vi "LabVIEW OPC UA Client.vi"() -> ()   [LabVIEW 2020]
uses:
  <vilib>/OPCUA/NI OPC UA Client.lvlib
  <vilib>/OPCUA/NI OPC UA Utility.lvlib
  <vilib>/OPCUA/controls/Write Status.ctl
  <vilib>/OPCUA/controls/NodeId.ctl
  <vilib>/OPCUA/client/Multiple Write Double.vi
  <vilib>/OPCUA/client/Multiple Read Double.vi
panel:
  out "DateTime":string
  out "Status":u32(ring) items=["Good", "Good_SubscriptionTransferred", "Good_CompletesAsynchronously", "Good_Overload", "Good_Clamped", "Good_LocalOverride", "Good_EntryInserted", "Good_EntryReplaced", "Good_NoData", "Good_MoreData", "Good_CommunicationEvent", "Good_ShutdownEvent", "Good_CallAgain", "Good_NonCriticalTimeout", "Good_ResultsMayBeIncomplete", "Good_DataIgnored", "Uncertain", "Uncertain_ReferenceOutOfServer", "Uncertain_NoCommunicationLastUsableValue", "Uncertain_LastUsableValue", "Uncertain_SubstituteValue", "Uncertain_InitialValue", "Uncertain_SensorNotAccurate", "Uncertain_EngineeringUnitsExceeded", "Uncertain_SubNormal", "Uncertain_DataSubNormal", "Uncertain_ReferenceNotDeleted", "Uncertain_NotAllNodesAvailable", "Bad", "Bad_UnexpectedError", "Bad_InternalError", "Bad_OutOfMemory", "Bad_ResourceUnavailable", "Bad_CommunicationError", "Bad_EncodingError", "Bad_DecodingError", "Bad_EncodingLimitsExceeded", "Bad_UnknownResponse", "Bad_Timeout", "Bad_ServiceUnsupported", "Bad_Shutdown", "Bad_ServerNotConnected", "Bad_ServerHalted", "Bad_NothingToDo", "Bad_TooManyOperations", "Bad_DataTypeIdUnknown", "Bad_CertificateInvalid", "Bad_SecurityChecksFailed", "Bad_CertificateTimeInvalid", "Bad_CertificateIssuerTimeInvalid", "Bad_CertificateHostNameInvalid", "Bad_CertificateUriInvalid", "Bad_CertificateUseNotAllowed", "Bad_CertificateIssuerUseNotAllowed", "Bad_CertificateUntrusted", "Bad_CertificateRevocationUnknown", "Bad_CertificateIssuerRevocationUnknown", "Bad_CertificateRevoked", "Bad_CertificateIssuerRevoked", "Bad_UserAccessDenied", "Bad_IdentityTokenInvalid", "Bad_IdentityTokenRejected", "Bad_SecureChannelIdInvalid", "Bad_InvalidTimestamp", "Bad_NonceInvalid", "Bad_SessionIdInvalid", "Bad_SessionClosed", "Bad_SessionNotActivated", "Bad_SubscriptionIdInvalid", "Bad_RequestHeaderInvalid", "Bad_TimestampsToReturnInvalid", "Bad_RequestCancelledByClient", "Bad_NoCommunication", "Bad_WaitingForInitialData", "Bad_NodeIdInvalid", "Bad_NodeIdUnknown", "Bad_AttributeIdInvalid", "Bad_IndexRangeInvalid", "Bad_IndexRangeNoData", "Bad_DataEncodingInvalid", "Bad_DataEncodingUnsupported", "Bad_NotReadable", "Bad_NotWritable", "Bad_OutOfRange", "Bad_NotSupported", "Bad_NotFound", "Bad_ObjectDeleted", "Bad_NotImplemented", "Bad_MonitoringModeInvalid", "Bad_MonitoredItemIdInvalid", "Bad_MonitoredItemFilterInvalid", "Bad_MonitoredItemFilterUnsupported", "Bad_FilterNotAllowed", "Bad_StructureMissing", "Bad_EventFilterInvalid", "Bad_ContentFilterInvalid", "Bad_FilterOperandInvalid", "Bad_ContinuationPointInvalid", "Bad_NoContinuationPoints", "Bad_ReferenceTypeIdInvalid", "Bad_BrowseDirectionInvalid", "Bad_NodeNotInView", "Bad_ServerUriInvalid", "Bad_ServerNameMissing", "Bad_DiscoveryUrlMissing", "Bad_SempahoreFileMissing", "Bad_RequestTypeInvalid", "Bad_SecurityModeRejected", "Bad_SecurityPolicyRejected", "Bad_TooManySessions", "Bad_UserSignatureInvalid", "Bad_ApplicationSignatureInvalid", "Bad_NoValidCertificates", "Bad_RequestCancelledByRequest", "Bad_ParentNodeIdInvalid", "Bad_ReferenceNotAllowed", "Bad_NodeIdRejected", "Bad_NodeIdExists", "Bad_NodeClassInvalid", "Bad_BrowseNameInvalid", "Bad_BrowseNameDuplicated", "Bad_NodeAttributesInvalid", "Bad_TypeDefinitionInvalid", "Bad_SourceNodeIdInvalid", "Bad_TargetNodeIdInvalid", "Bad_DuplicateReferenceNotAllowed", "Bad_InvalidSelfReference", "Bad_ReferenceLocalOnly", "Bad_NoDeleteRights", "Bad_ServerIndexInvalid", "Bad_ViewIdUnknown", "Bad_TooManyMatches", "Bad_QueryTooComplex", "Bad_NoMatch", "Bad_MaxAgeInvalid", "Bad_HistoryOperationInvalid", "Bad_HistoryOperationUnsupported", "Bad_WriteNotSupported", "Bad_TypeMismatch", "Bad_MethodInvalid", "Bad_ArgumentsMissing", "Bad_TooManySubscriptions", "Bad_TooManyPublishRequests", "Bad_NoSubscription", "Bad_SequenceNumberUnknown", "Bad_MessageNotAvailable", "Bad_InsufficientClientProfile", "Bad_TcpServerTooBusy", "Bad_TcpMessageTypeInvalid", "Bad_TcpSecureChannelUnknown", "Bad_TcpMessageTooLarge", "Bad_TcpNotEnoughResources", "Bad_TcpInternalError", "Bad_TcpEndpointUrlInvalid", "Bad_RequestInterrupted", "Bad_RequestTimeout", "Bad_SecureChannelClosed", "Bad_SecureChannelTokenUnknown", "Bad_SequenceNumberInvalid", "Bad_ConfigurationError", "Bad_NotConnected", "Bad_DeviceFailure", "Bad_SensorFailure", "Bad_OutOfService", "Bad_DeadbandFilterInvalid", "Bad_RefreshInProgress", "Bad_ConditionAlreadyDisabled", "Bad_ConditionDisabled", "Bad_EventIdUnknown", "Bad_NoData", "Bad_DataLost", "Bad_DataUnavailable", "Bad_EntryExists", "Bad_NoEntryExists", "Bad_TimestampNotSupported", "Bad_InvalidArgument", "Bad_ConnectionRejected", "Bad_Disconnect", "Bad_ConnectionClosed", "Bad_InvalidState", "Bad_EndOfStream", "Bad_NoDataAvailable", "Bad_WaitingForResponse", "Bad_OperationAbandoned", "Bad_ExpectedStreamToBlock", "Bad_WouldBlock", "Bad_SyntaxError", "Bad_MaxConnectionsReached", "Bad_RequestTooLarge", "Bad_ResponseTooLarge", "Bad_EventNotAcknowledgeable", "Bad_InvalidTimestampArgument", "Bad_ProtocolVersionUnsupported", "Bad_StateNotActive", "Bad_FilterOperatorInvalid", "Bad_FilterOperatorUnsupported", "Bad_FilterOperandCountMismatch", "Bad_FilterElementInvalid", "Bad_FilterLiteralInvalid", "Bad_IdentityChangeNotSupported", "Bad_NotTypeDefinition", "Bad_ViewTimestampInvalid", "Bad_ViewParameterMismatch", "Bad_ViewVersionInvalid", "Bad_ConditionAlreadyEnabled", "Bad_DialogNotActive", "Bad_DialogResponseInvalid", "Bad_ConditionBranchAlreadyAcked", "Bad_ConditionBranchAlreadyConfirmed", "Bad_ConditionAlreadyShelved", "Bad_ConditionNotShelved", "Bad_ShelvingTimeOutOfRange", "Bad_AggregateListMismatch", "Bad_AggregateNotSupported", "Bad_AggregateInvalidInputs", "Bad_BoundNotFound", "Bad_BoundNotSupported", "Bad_AggregateConfigurationRejected", "Bad_TooManyMonitoredItems"]
  in  "NodeId":string(combo)
  out "Connected":bool
  in  "Server Address":string
  in  "Write Button":bool
  out "Value":dbl
  in  "New Value":dbl
  in  "Disconnect Button":bool
  in  "Connect Button":bool
  out "Error out":errorcluster
  in  "Error in":errorcluster
  in  "Exit Button":bool
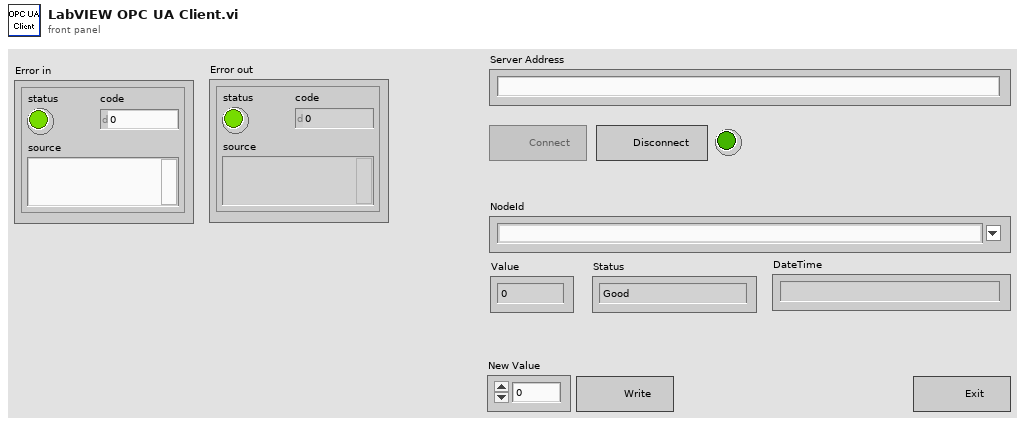
[diagram p1: front panel]
types:
  T1 = enum8{"Enabled", "Disabled", "Disabled and Grayed Out"}
  T2 = cluster{"message mode":enum16{"None", "Sign", "Sign and Encrypt"}, "security":enum16{"Basic256", "Basic128Rsa15"}}
  T3 = typedef "OPC UA Client Refnum.ctl" = refnum<k21>
  T4 = typedef "NodeId.ctl" = string
  T5 = typedef "OPC UA StatusCode.ctl" = u32
  T6 = cluster{"node ID":T4, "value ":dbl, "timestamp":timestamp, "status":T5}[]
  T7 = cluster{"node ID":T4, "value ":dbl, "timestamp":timestamp, "status":T5}
  T8 = typedef "Write Status.ctl" = u32
  T9 = cluster{"node ID":T4, "value":dbl, "timestamp (current time)":timestamp, "node status":T8}
  T10 = cluster{"node ID":T4, "value":dbl, "timestamp (current time)":timestamp, "node status":T8}[]
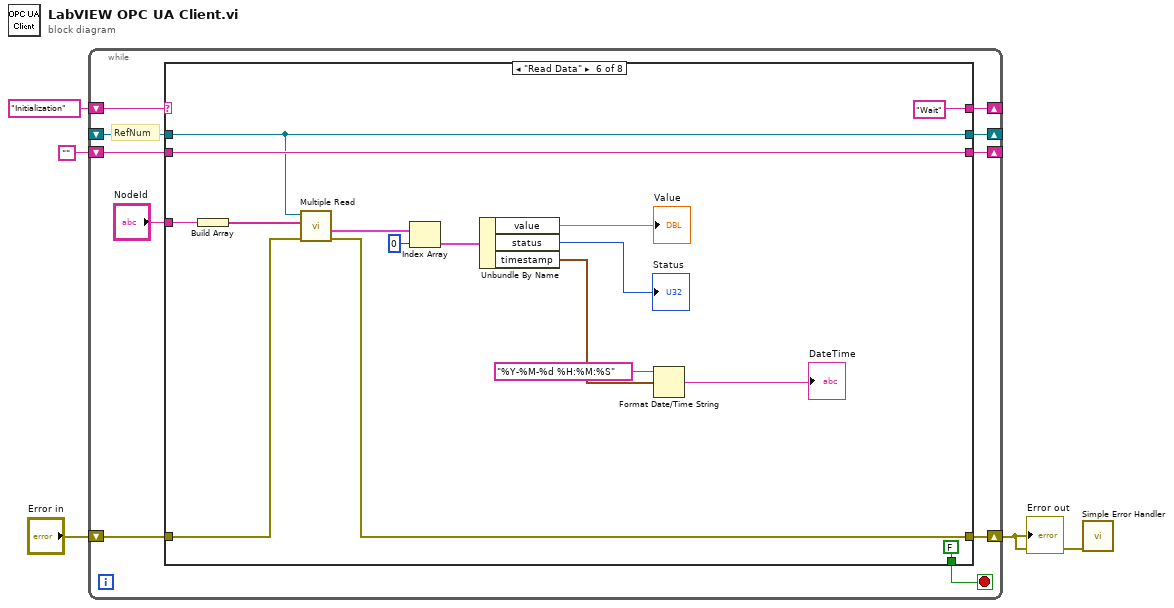
[diagram p0: block diagram]
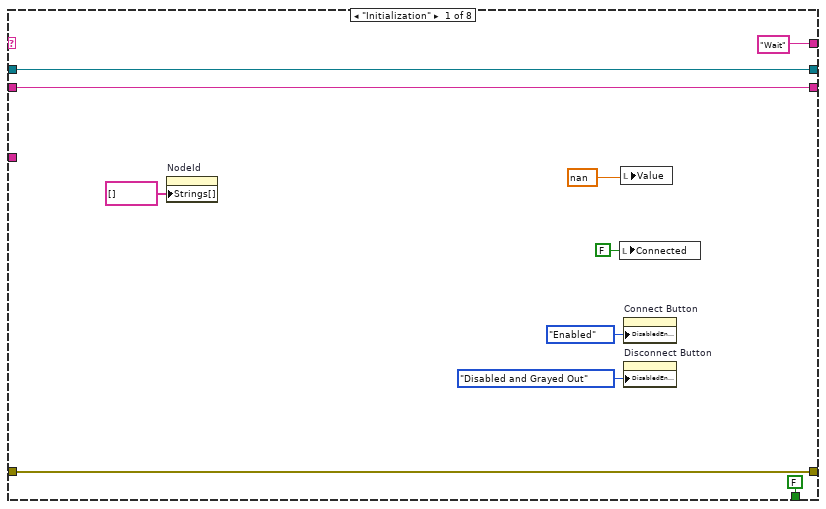
[diagram p2: hidden frame]
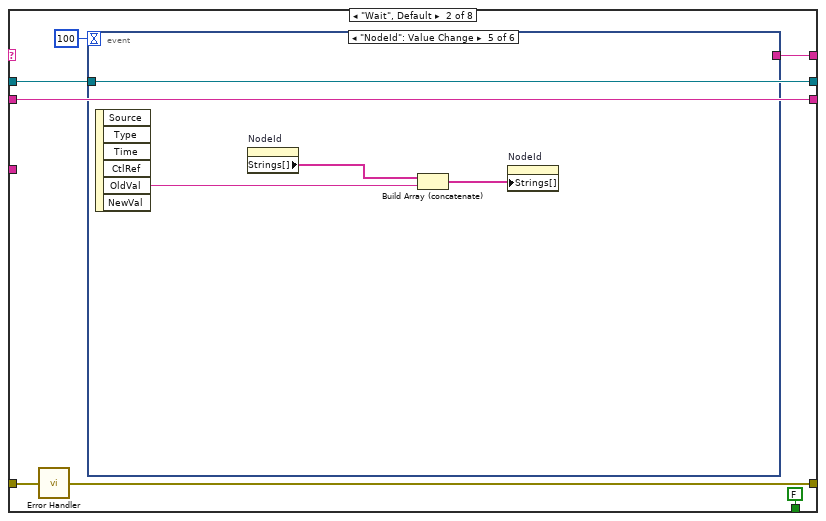
[diagram p3: hidden frame]
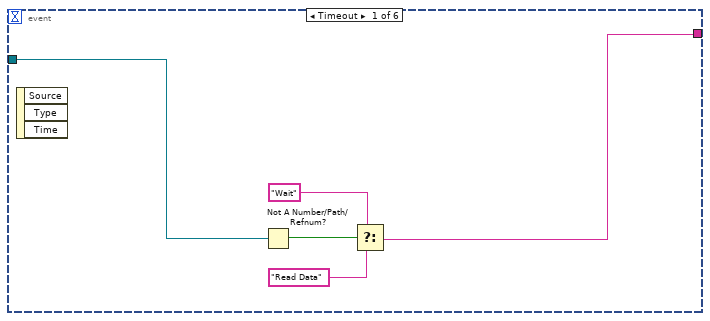
[diagram p4: hidden frame]
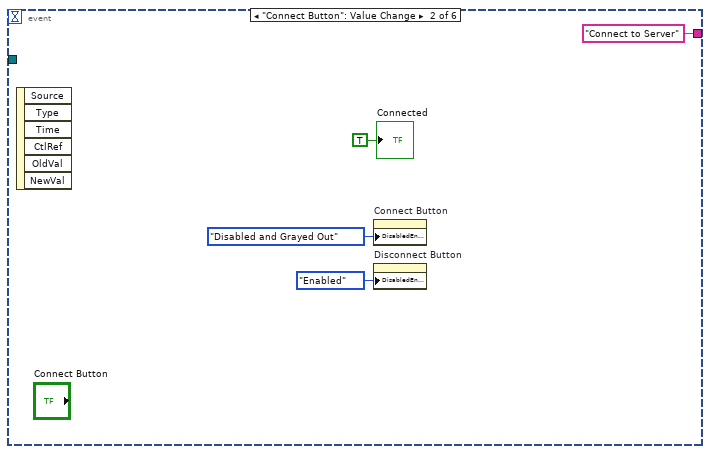
[diagram p5: hidden frame]
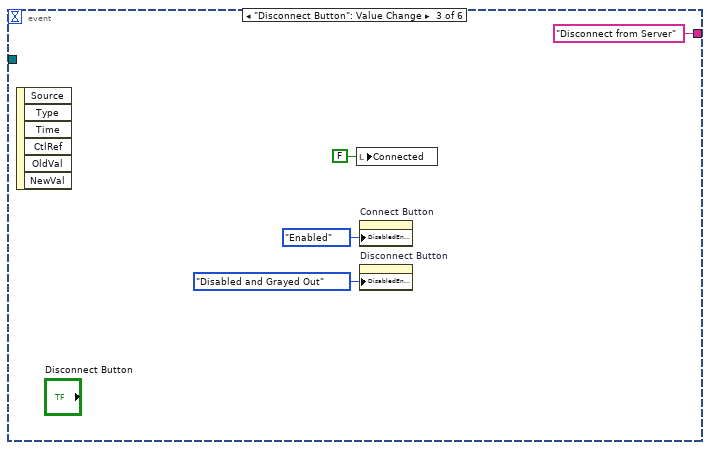
[diagram p6: hidden frame]
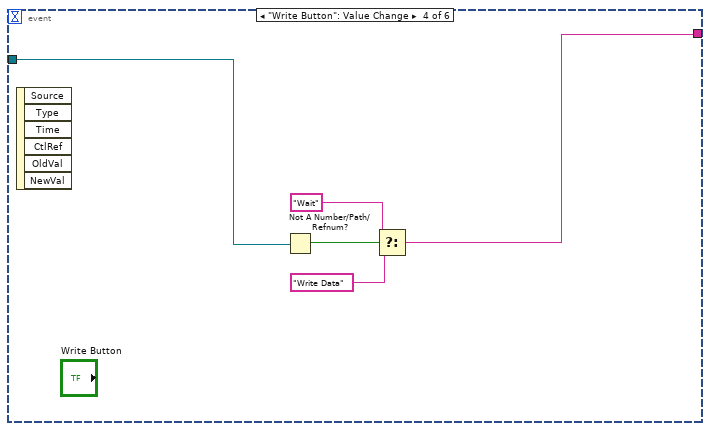
[diagram p7: hidden frame]
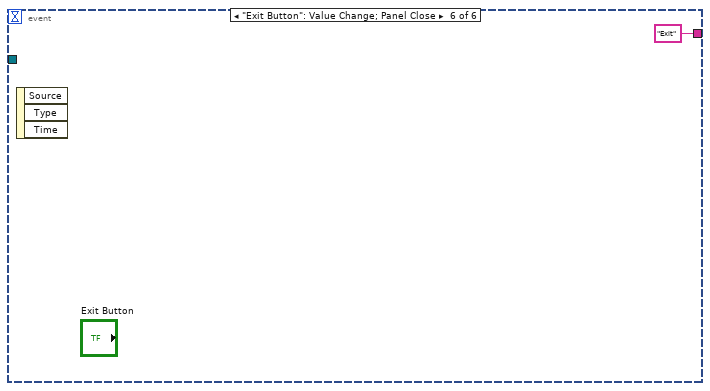
[diagram p8: hidden frame]
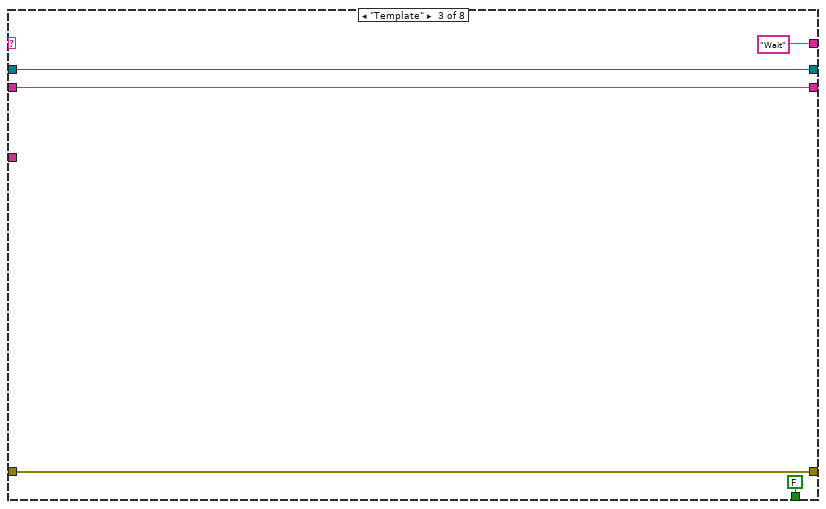
[diagram p9: hidden frame]
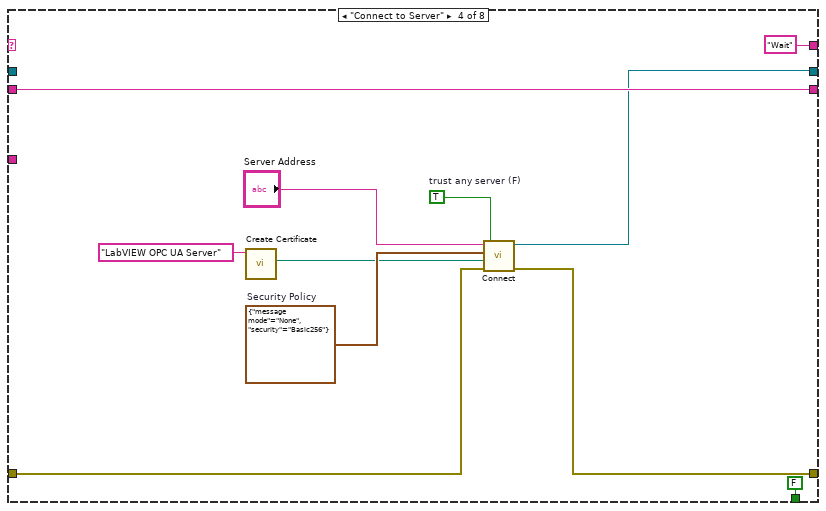
[diagram p10: hidden frame]
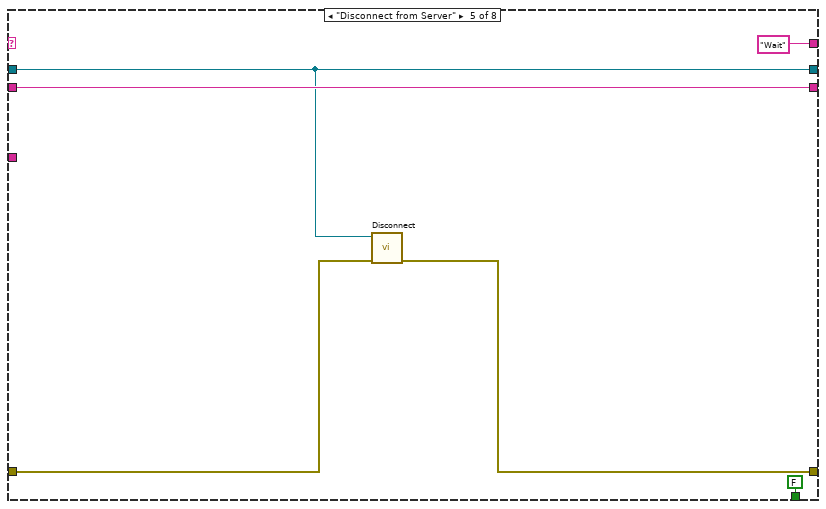
[diagram p11: hidden frame]
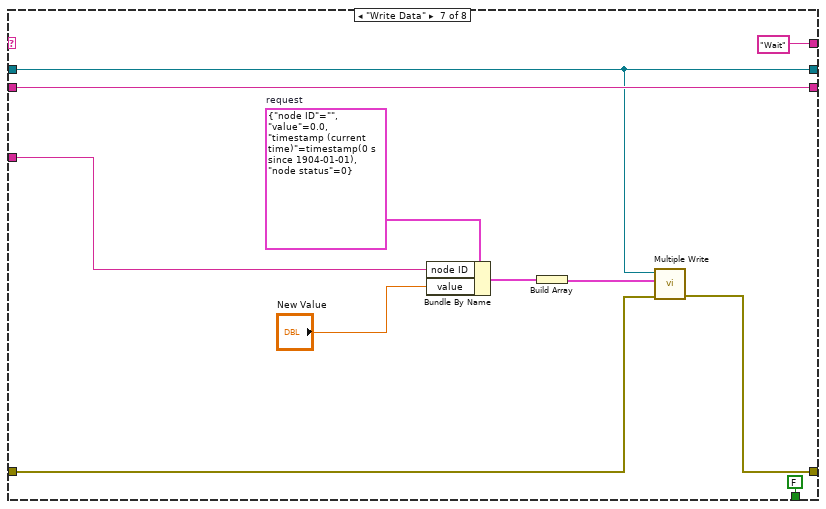
[diagram p12: hidden frame]
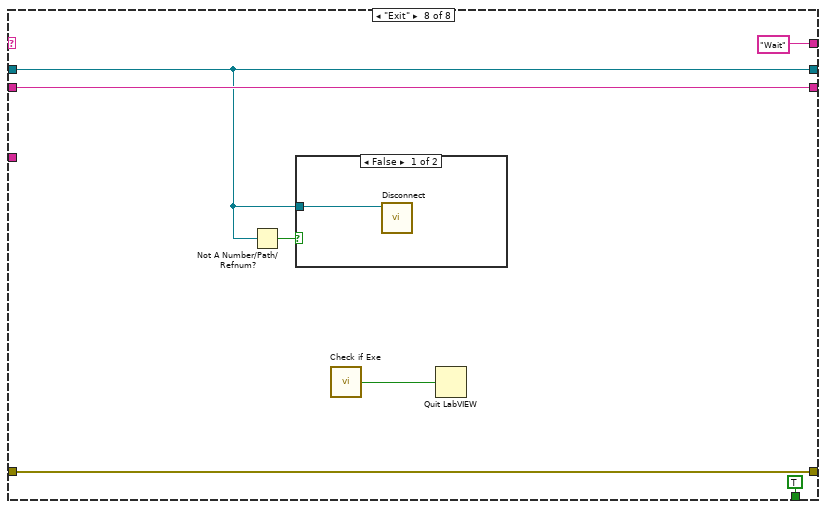
[diagram p13: hidden frame]
diagram:
  n1 = while {
    shift-right: [w13] -> _
    shift-left: "Initialization" -> [w14]
    shift-right: [w11] -> _
    shift-left: _ -> [w10]
    shift-right: [w9] -> w2
    shift-left: "Error in" -> [w8]
    shift-right: [w7] -> _
    shift-left: "" -> [w6]
    stop <- w12 stop-if-true
    # "RefNum"
    n2 = case shown="\"Read Data\"" w14 {
      tunnel: ["Wait" w31 "Wait" "Wait" "Wait" "Wait" "Wait" "Wait"] -> w13
      tunnel: [FALSE FALSE FALSE FALSE FALSE FALSE FALSE TRUE] -> w12
      tunnel: [w22 w27 w56 w62 w72 w83 w92 w103] -> w11
      tunnel: w10 -> [w22 w27 w56 _ w72 w83 w92 w103]
      tunnel: [w21 w26 w55 w61 w71 w81 w94 w107] -> w9
      tunnel: w8 -> [w21 w25 w55 w60 w70 w80 w93 w107]
      tunnel: [w20 w28 w54 w67 w73 w89 w100 w104] -> w7
      tunnel: w6 -> [w20 w28 w54 w67 w73 w89 w100 w104]
      tunnel: "NodeId" -> [_ _ _ _ _ w84 w96 _]
      frame "Initialization" {
        n3 = property on="NodeId" class="CmbBox"("Strings[]"=string[] [] ("Strings []")) -> ()  [unwired: 2 in, 2 out]
        n4 = local write "Connected"(FALSE ("Connected")) -> ()
        n5 = local write "Value"(nan) -> ()
        n6 = property on="Connect Button" class="Bool"("DisabledEnum"=T1."Enabled" ("Disabled")) -> ()  [unwired: 2 in, 2 out]
        n7 = property on="Disconnect Button" class="Bool"("DisabledEnum"=T1."Disabled and Grayed Out" ("Disabled")) -> ()  [unwired: 2 in, 2 out]
      }
      frame "Wait", Default {
        n8 = call "Error Handler.vi"("Error in"=w25) -> ("Error out"=w26:errorcluster)
        n9 = event shown="[4] \"NodeId\": Value Change" {
          selector: _ -> [_ _ _ _ _ _]
          dyn-events: _ -> [_ _ _ _ _ _]
          timeout: 100 -> [_ _ _ _ _ _]
          tunnel: [w33 "Connect to Server" "Disconnect from Server" w46 _ "Exit"] -> w31
          tunnel: w27 -> [w32 _ _ w45 _ _]
          event Timeout {
            n10 = event-data() -> ()  [unwired: 1 in, 3 out]
            n11 = Not A Number/Path/Refnum?(number/path/refnum=w32) -> (NaN/Path/Refnum?=w36:bool)
            n12 = Select(t="Wait", s=w36, f="Read Data") -> (s? t:f=w33:string)
          }
          event "Connect Button": Value Change {
            n13 = event-data() -> ()  [unwired: 1 in, 6 out]
            n14 = property on="Connect Button" class="Bool"("DisabledEnum"=T1."Disabled and Grayed Out" ("Disabled")) -> ()  [unwired: 2 in, 2 out]
            n15 = property on="Disconnect Button" class="Bool"("DisabledEnum"=T1."Enabled" ("Disabled")) -> ()  [unwired: 2 in, 2 out]
            "Connected" <- TRUE ("Connected")
          }
          event "Disconnect Button": Value Change {
            n16 = event-data() -> ()  [unwired: 1 in, 6 out]
            n17 = local write "Connected"(FALSE ("Connected")) -> ()
            n18 = property on="Connect Button" class="Bool"("DisabledEnum"=T1."Enabled" ("Disabled")) -> ()  [unwired: 2 in, 2 out]
            n19 = property on="Disconnect Button" class="Bool"("DisabledEnum"=T1."Disabled and Grayed Out" ("Disabled")) -> ()  [unwired: 2 in, 2 out]
          }
          event "Write Button": Value Change {
            n20 = event-data() -> ()  [unwired: 1 in, 6 out]
            n21 = Not A Number/Path/Refnum?(number/path/refnum=w45) -> (NaN/Path/Refnum?=w49:bool)
            n22 = Select(t="Wait", s=w49, f="Write Data") -> (s? t:f=w46:string)
          }
          event "NodeId": Value Change {
            n23 = event-data() -> ("OldVal"=w51:string)  [unwired: 1 in, 5 out]
            n24 = property on="NodeId" class="CmbBox"() -> ("Strings[]"=w52:string[])  [unwired: 2 in, 2 out]
            n25 = Build Array (concatenate) "Build Array"(w52, w51) -> (w50:string[])
            n26 = property on="NodeId" class="CmbBox"("Strings[]"=w50) -> ()  [unwired: 2 in, 2 out]
          }
          event "Exit Button": Value Change; Panel Close {
            n27 = event-data() -> ()  [unwired: 1 in, 3 out]
          }
        }
      }
      frame "Template" {
      }
      frame "Connect to Server" {
        w59 = TRUE  # trust any server (F)
        w66 = T2 {"message mode"=enum."None", "security"=enum."Basic256"}  # Security Policy
        n28 = call <vilib>:"Create Certificate.vi"("certificate name in"="LabVIEW OPC UA Server") -> ("certificate path"=w64:path)  [unwired: 7 in, 3 out]
        n29 = call <vilib>:"Connect.vi"("trust any server (F)"=w59, "error in (no error)"=w60, "client certificate file"=w64, "security policy"=w66, "server endpoint URL"="Server Address") -> ("error out"=w61:errorcluster, "OPC UA client refnum out"=w62:T3)  [unwired: 4 in, 1 out]
      }
      frame "Disconnect from Server" {
        n30 = call <vilib>:"Disconnect.vi"("error in (no error)"=w70, "OPC UA client refnum in"=w72) -> ("error out"=w71:errorcluster)  [unwired: 9 in]
      }
      frame "Read Data" {
        n31 = Build Array "Build Array"(w84) -> (w88:string[])
        n32 = call-poly <vilib>:"Multiple Read.vi"("error in (no error)"=w80, "node IDs"=w88, "OPC UA client refnum in"=w83) -> ("error out"=w81:errorcluster, "results"=w87:T6)  [unwired: 5 in, 2 out]
        n33 = Index Array "Index Array"(array=w87, index=0) -> (element=w85:T7)
        n34 = Unbundle By Name "Unbundle By Name"(w85) -> ("value"=→"Value":dbl, "status"=→"Status":T5, "timestamp"=w78:timestamp)
        n35 = Format Date/Time String(time format string (%c)="%Y-%M-%d %H:%M:%S", seconds (now)=w78) -> (date/time string=→"DateTime":string)  [unwired: 1 in]
      }
      frame "Write Data" {
        w99 = T9 {"node ID"="", "value"=0.0, "timestamp (current time)"=timestamp(0 s since 1904-01-01), "node status"=0}  # request
        n36 = Bundle By Name "Bundle By Name"(cluster=w99, "node ID"=w96, "value"="New Value") -> (w97:T9)
        n37 = Build Array "Build Array"(w97) -> (w98:T10)
        n38 = call-poly <vilib>:"Multiple Write.vi"("error in (no error)"=w93, "requests"=w98, "OPC UA client refnum in"=w92) -> ("error out"=w94:errorcluster)  [unwired: 5 in, 3 out]
      }
      frame "Exit" {
        n39 = Not A Number/Path/Refnum?(number/path/refnum=w103) -> (NaN/Path/Refnum?=w105:bool)
        n40 = case shown="False" w105 {
          tunnel: w103 -> [w110 _]
          frame False {
            n41 = call <vilib>:"Disconnect.vi"("OPC UA client refnum in"=w110) -> ()  [unwired: 10 in, 1 out]
          }
          frame True {
          }
        }
        n42 = call "Check if Exe.vi"() -> ("Executable Application?"=w106:bool)  [unwired: 1 in]
        n43 = Quit LabVIEW(quit? (T)=w106) -> ()
      }
    }
  }
  "Error out" <- w2
  n44 = call <vilib>:"Simple Error Handler.vi"("error in (no error)"=w2) -> ()  [unwired: 4 in, 5 out]
